vi "Scratch.vi"() -> ()   [LabVIEW 2020]
uses:
  obs-websocket/OBS/OBS.lvclass
  obs-websocket/Input Settings.ctl
  obs-websocket/obs-websocket.lvlib
  obs-websocket/Input.ctl
panel:
  out "Input Kinds":string[](array[string])
  out "Inputs":T1[](array[typedef])
  in  "Password":string="44S4aN6PpCHpVM4Y"
  out "Program Scene":string
  out "Preview Image":picture
  out "error out":errorcluster
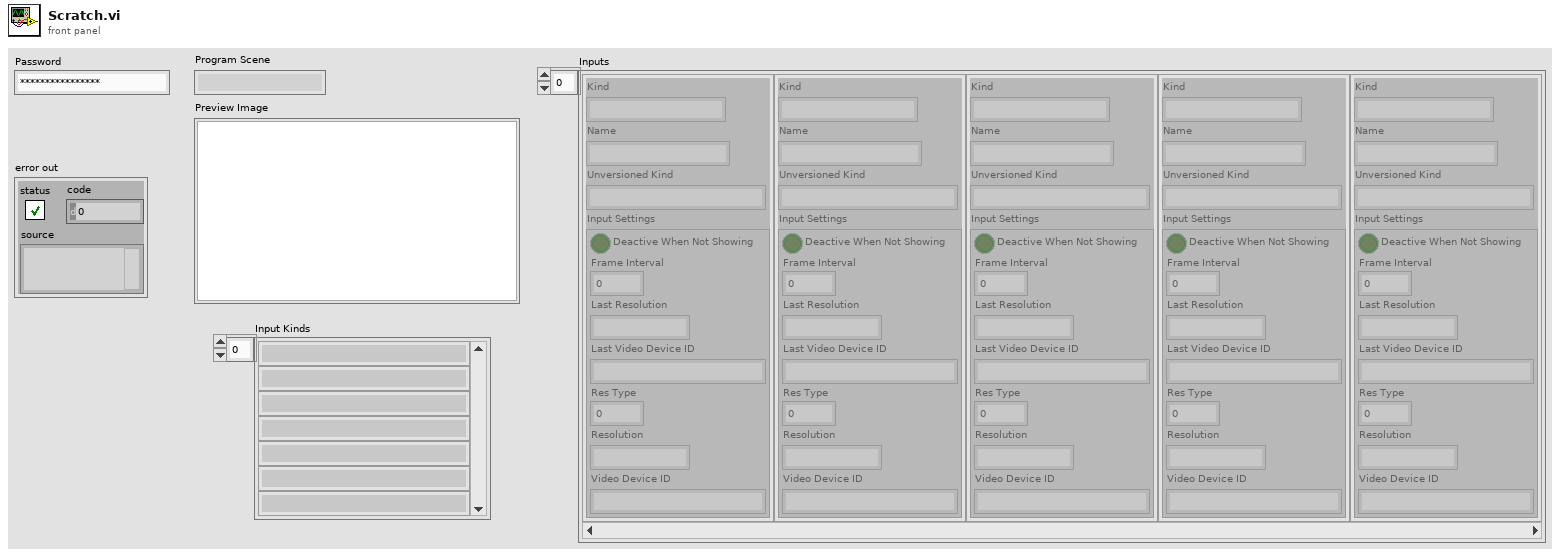
[diagram p1: front panel]
types:
  T1 = typedef "obs-websocket.lvlib/Input.ctl" = cluster{"Kind":string, "Name":string, "Unversioned Kind":string, "Input Settings":T2}
  T2 = typedef "obs-websocket.lvlib/Input Settings.ctl" = cluster{"Deactive When Not Showing":bool, "Frame Interval":i32, "Last Resolution":string, "Last Video Device ID":string, "Res Type":i32, "Resolution":string, "Video Device ID":string}
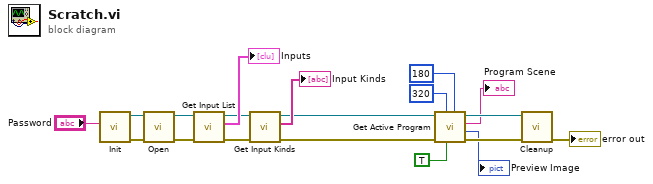
[diagram p0: block diagram]
diagram:
  n1 = call "Init.vi"("Password (None)"="Password") -> ("error out"=w18:errorcluster, "OBS out"=w19:refnum<class "OBS.lvclass">)  [unwired: 9 in]
  n2 = call "Open.vi"("error in (no error)"=w18, "OBS in"=w19) -> ("error out"=w7:errorcluster, "OBS out"=w8:refnum<class "OBS.lvclass">)  [unwired: 8 in]
  n3 = call "Get Input List.vi"("error in (no error)"=w7, "OBS in"=w8) -> ("error out"=w4:errorcluster, "Inputs"=→"Inputs":T1[], "OBS out"=w5:refnum<class "OBS.lvclass">)  [unwired: 7 in]
  n4 = call "Get Input Kinds.vi"("error in (no error)"=w4, "OBS in"=w5) -> ("error out"=w1:errorcluster, "Input Kinds"=→"Input Kinds":string[], "OBS out"=w2:refnum<class "OBS.lvclass">)  [unwired: 7 in]
  n5 = call "Get Active Program.vi"("Preview Height (Source)"=180 ("Preview Width (Source)"), "Get Preview Image? (F)"=TRUE, "Preview Width (Source)"=320, "error in (no error)"=w1, "OBS in"=w2) -> ("error out"=w14:errorcluster, "Preview Image"=→"Preview Image":picture, "Program Scene"=→"Program Scene":string, "OBS out"=w15:refnum<class "OBS.lvclass">)  [unwired: 3 in]
  n6 = call "Cleanup.vi"("error in (no error)"=w14, "OBS in"=w15) -> ("error out"=→"error out":errorcluster)  [unwired: 9 in]
